vi "visn_Calculate CRC-5 (Bits Array)Fer2.vi"(11 "Bits Array":u8[](array[numeric])=[1, 1, 0, 0, 1, 1, 1, 0, 1, 0] format="%0x") -> (3 "CRC-5":u8[](array[numeric])=[1, 0, 0, 0, 0] format="%0x")   [LabVIEW 2015]
panel:
  out "loop":i32
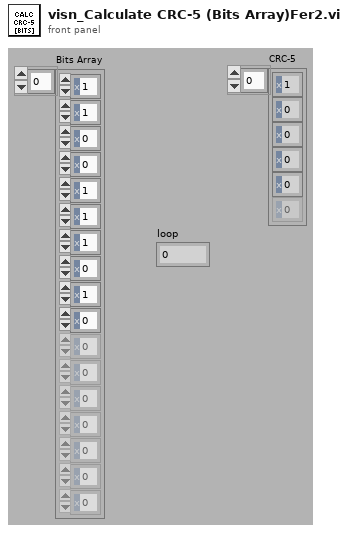
[diagram p1: front panel]
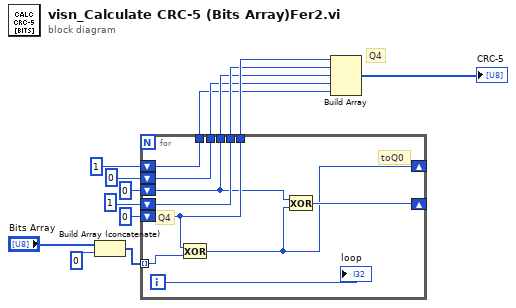
[diagram p0: block diagram]
diagram:
  # "Q4"
  n1 = Build Array (concatenate)("Bits Array", u8 0) -> (w8:u8[])
  n2 = for {
    tunnel: w8 -> [w22] mode=indexing
    tunnel: [w21] -> w14
    tunnel: [w20] -> w13
    tunnel: [w15] -> w12
    tunnel: [w19] -> w11
    tunnel: [w18] -> w10
    shift-right: [w16] -> _
    shift-left: u8 1 -> [w18]
    shift-left: u8 0 -> [w19]
    shift-left: u8 0 -> [w15]
    shift-right: [w17] -> _
    shift-left: u8 1 -> [w20]
    shift-left: u8 0 -> [w21]
    i -> [w23]
    # "toQ0"
    # "Q4"
    n3 = Exclusive Or(1:w22, 2:w21) -> (0:w16:u8)
    n4 = Exclusive Or(1:w16, 2:w15) -> (0:w17:u8)
    "loop" <- w23
  }
  n5 = Build Array(w14, w13, w12, w11, w10) -> (→"CRC-5":u8[])
